vi "CODMn质控流程 (子VI).vi"(9 "CODMn量程切换":enum32{"H", "L", "AUTO"}(ring)=enum."AUTO", 10 "CODMn":bool) -> (3 "布尔":bool)   [LabVIEW 2016, in "质控单元.lvlib"]
panel:
  out "CODMn中断报警":bool
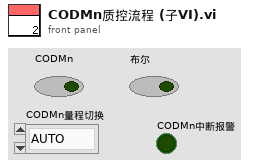
[diagram p1: front panel]
types:
  T1 = enum16{"待机", "启动水样测量", "水样测量中", "启动加标", "启动加标回收", "加标回收测量中", "结束"}
  T2 = cluster{"测量模式":enum16{"水样测量", "标样核查", "零点核查", "跨度核查", "空白测试", "加标回收", "平行样", "校零", "校标"}}
  T3 = enum16{"空闲", "水样测试", "标样核查", "零点核查", "跨度核查", "空白测试", "平行样测试", "质控样", "空白校准", "标样校准", "加标回收"}
  T4 = enum16{"空闲", "水样测试", "标样核查", "零点核查", "跨度核查", "空白测试", "平行样测试", "加标回收", "空白校准", "标样校准", "初始化（清洗）"}
  T5 = cluster{"量程":dbl, "检出限":dbl, "加标前水样浓度":dbl, "加标后水样浓度":dbl, "加标水杯定容体积":dbl, "加标母液浓度":dbl, "加标体积":dbl, "加标回收率":dbl}
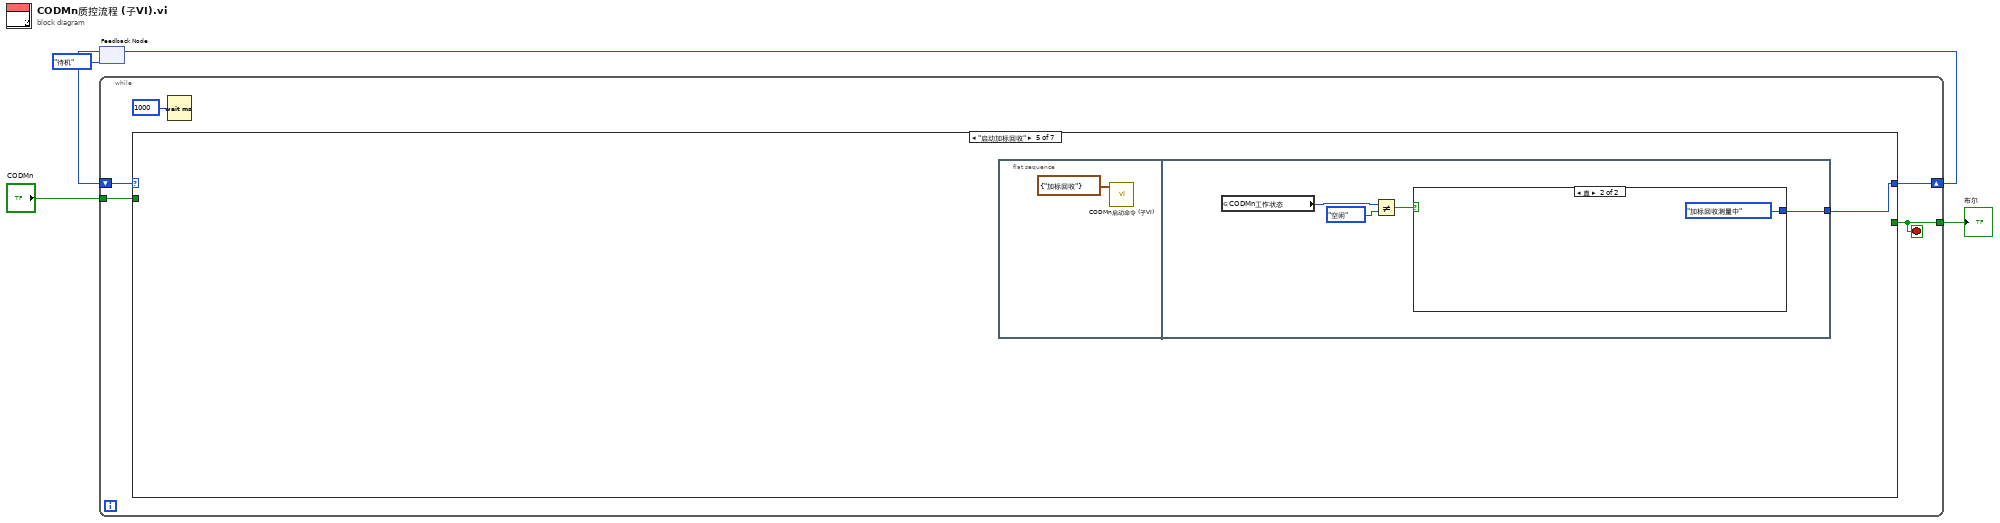
[diagram p0: block diagram]
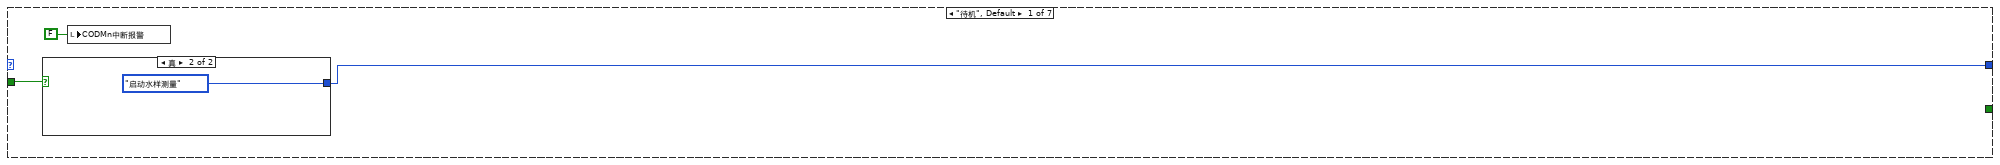
[diagram p2: hidden frame]
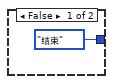
[diagram p3: hidden frame]
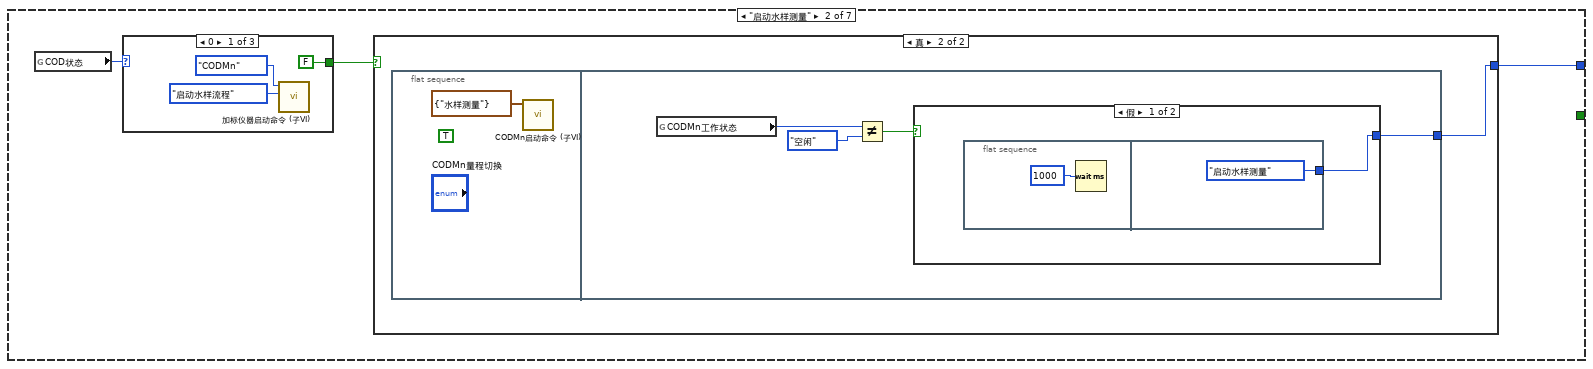
[diagram p4: hidden frame]
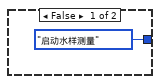
[diagram p5: hidden frame]
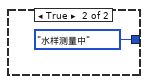
[diagram p6: hidden frame]
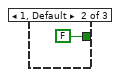
[diagram p7: hidden frame]
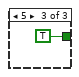
[diagram p8: hidden frame]
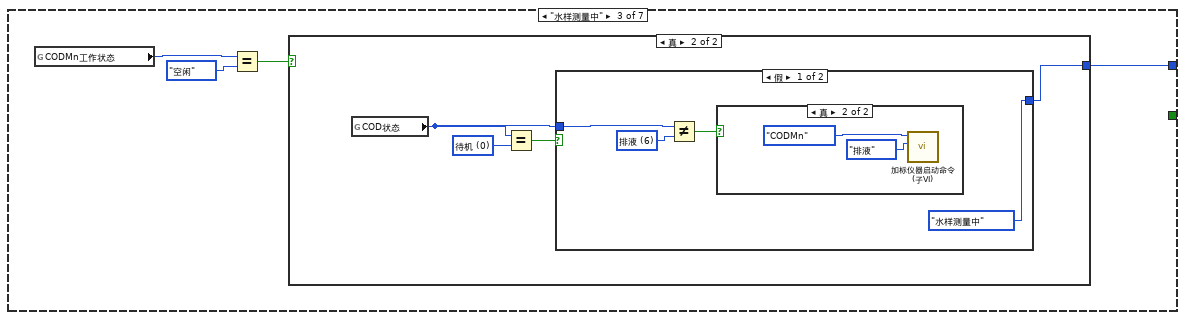
[diagram p9: hidden frame]
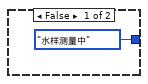
[diagram p10: hidden frame]
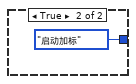
[diagram p12: hidden frame]
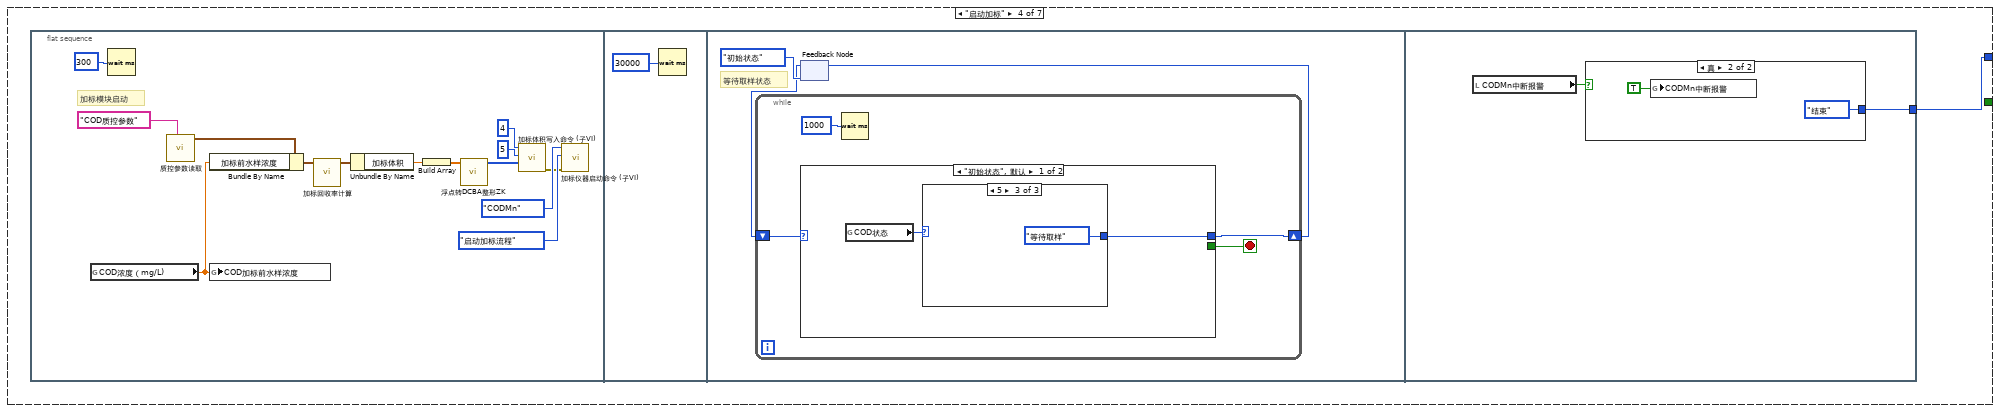
[diagram p13: hidden frame]
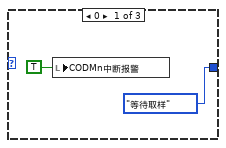
[diagram p14: hidden frame]
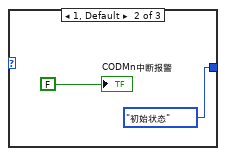
[diagram p15: hidden frame]
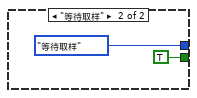
[diagram p16: hidden frame]
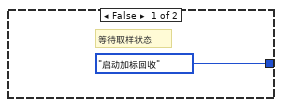
[diagram p17: hidden frame]
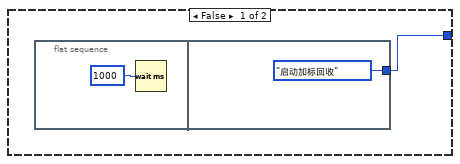
[diagram p18: hidden frame]
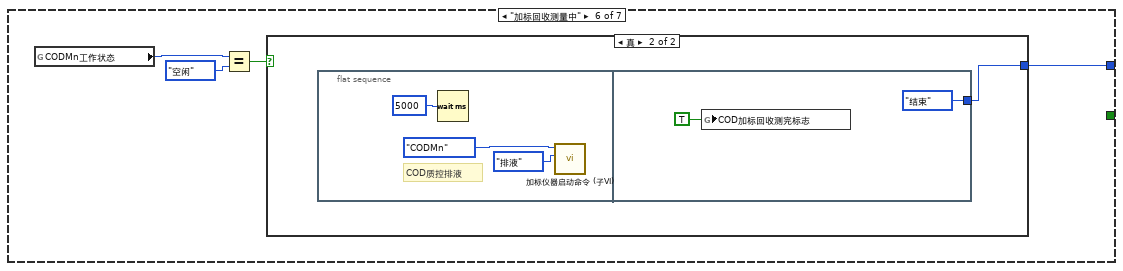
[diagram p19: hidden frame]
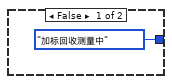
[diagram p20: hidden frame]
diagram:
  n1 = feedback #1(T1."待机") -> (w1:T1)
  n2 = while {
    tunnel: "CODMn" -> [w10]
    tunnel: [w6] -> w3
    shift-right: [w9] -> w4
    shift-left: w1 -> [w8]
    stop <- w6 stop-if-true
    n3 = case shown="\"启动加标回收\"" w8 {
      tunnel: [w13 w18 w38 w51 w88 w101 T1."结束"] -> w9
      tunnel: [_ _ _ _ _ _ TRUE] -> w6
      tunnel: w10 -> [w12 _ _ _ _ _ _]
      frame "待机", Default {
        n4 = case shown="真" w12 {
          tunnel: [T1."结束" T1."启动水样测量"] -> w13
          frame False {
          }
          frame True {
          }
        }
        n5 = local write "CODMn中断报警"(FALSE ("CODMn中断报警")) -> ()
      }
      frame "启动水样测量" {
        n6 = global read "加标回收状态全局变量.vi" "COD状态"() -> (w17:u16)
        n7 = case shown="0" w17 {
          tunnel: [FALSE ("s") FALSE ("s") TRUE ("s")] -> w16
          frame 0 {
            n8 = call "加标仪器启动命令 (子VI).vi"("启动命令"=enum16{"启动水样流程", "启动加标流程", "排液", "停止"}."启动水样流程", "仪器"=enum16{"", "氨氮", "总磷", "总氮", "CODMn", "CODCr"}."CODMn") -> ()  [unwired: 9 in, 1 out]
          }
          frame 1, Default {
          }
          frame 5 {
          }
        }
        n9 = case shown="真" w16 {
          tunnel: [T1."启动水样测量" w20] -> w18
          frame False {
          }
          frame True {
            n10 = flat-sequence {
              tunnel: [w25] -> w20
              frame #0 {
                (unwired) TRUE ("强制切换")
                n11 = call "CODMn启动命令 (子VI).vi"("启动测量模式"=T2 {"测量模式"=enum."水样测量"}) -> ()  [unwired: 10 in, 1 out]
              }
              frame #1 {
                n12 = global read "与CODMn交互全局.vi" "CODMn工作状态"() -> (w24:T4)
                n13 = Not Equal?(x=w24, y=T3."空闲") -> (x != y?=w22:bool)
                n14 = case shown="假" w22 {
                  tunnel: [w26 T1."水样测量中"] -> w25
                  frame False {
                    n15 = flat-sequence {
                      tunnel: [T1."启动水样测量"] -> w26
                      frame #0 {
                        n16 = Wait (ms)(milliseconds to wait=u32 1000 ("等待时间（毫秒）")) -> ()  [unwired: 1 out]
                      }
                      frame #1 {
                      }
                    }
                  }
                  frame True {
                  }
                }
              }
            }
          }
        }
      }
      frame "水样测量中" {
        n17 = global read "与CODMn交互全局.vi" "CODMn工作状态"() -> (w37:T4)
        n18 = Equal?(x=w37, y=T3."空闲") -> (x = y?=w35:bool)
        n19 = case shown="真" w35 {
          tunnel: [T1."水样测量中" w43] -> w38
          frame False {
          }
          frame True {
            w42 = u16 0 items=["待机", "润洗", "进样", "进样完成", "柱塞泵加标", "等待取液", "排液"] ("COD状态")
            n20 = global read "加标回收状态全局变量.vi" "COD状态"() -> (w40:u16)
            n21 = Equal?(x=w40, y=w42) -> (x = y?=w41:bool)
            n22 = case shown="假" w41 {
              tunnel: [T1."水样测量中" T1."启动加标"] -> w43
              tunnel: w40 -> [w45 _]
              frame False {
                w46 = u16 6 items=["待机", "润洗", "进样", "进样完成", "柱塞泵加标", "等待取液", "排液"] ("氨氮状态")
                n23 = Not Equal?(x=w45, y=w46) -> (x != y?=w44:bool)
                n24 = case shown="真" w44 {
                  frame False {
                  }
                  frame True {
                    n25 = call "加标仪器启动命令 (子VI).vi"("启动命令"=enum16{"启动水样流程", "启动加标流程", "排液", "停止"}."排液", "仪器"=enum16{"", "氨氮", "总磷", "总氮", "CODMn", "CODCr"}."CODMn") -> ()  [unwired: 9 in, 1 out]
                  }
                }
              }
              frame True {
              }
            }
          }
        }
      }
      frame "启动加标" {
        n26 = flat-sequence {
          tunnel: [w84] -> w51
          frame #0 {
            # "加标模块启动"
            n27 = global read "与CODMn交互全局.vi" "COD浓度（mg/L)"() -> (w60:dbl)
            n28 = Wait (ms)(milliseconds to wait=u32 300 ("等待时间（毫秒）")) -> ()  [unwired: 1 out]
            n29 = call "质控参数读取.vi"("section"="COD质控参数") -> ("参数"=w63:T5)  [unwired: 9 in, 1 out]
            n30 = Bundle By Name(cluster=w63, "加标前水样浓度"=w60) -> (w64:T5)
            n31 = global write "水样浓度全局.vi" "COD加标前水样浓度"(w60) -> ()
            n32 = call "加标回收率计算.vi"("参数"=w64) -> ("参数 out"=w62:T5)  [unwired: 9 in, 1 out]
            n33 = Unbundle By Name(w62) -> ("加标体积"=w61:dbl)
            n34 = Build Array(w61) -> (w58:dbl[])
            n35 = call "浮点转DCBA整形ZK.vi"("浮点数"=w58) -> ("DCBA整形输出"=w53:u16[])  [unwired: 10 in]
            n36 = call "加标体积写入命令 (子VI).vi"("values"=w53, "starting address"=u16 5, "Slave ID"=u16 4 ("value")) -> ("错误输出"=w52:errorcluster)  [unwired: 8 in]
            n37 = call "加标仪器启动命令 (子VI).vi"("错误输入（无错误）"=w52, "启动命令"=enum16{"启动水样流程", "启动加标流程", "排液", "停止"}."启动加标流程", "仪器"=enum16{"", "氨氮", "总磷", "总氮", "CODMn", "CODCr"}."CODMn") -> ()  [unwired: 8 in, 1 out]
          }
          frame #1 {
            n38 = Wait (ms)(milliseconds to wait=u32 30000 ("等待时间（毫秒）")) -> ()  [unwired: 1 out]
          }
          frame #2 {
            # "等待取样状态"
            n39 = feedback #2(enum16{"初始状态", "等待取样"}."初始状态") -> (w68:enum16{"初始状态", "等待取样"})
            n40 = while {
              shift-right: [w72] -> w67
              shift-left: w68 -> [w73]
              stop <- w71 stop-if-true
              n41 = case shown="\"初始状态\", 默认" w73 {
                tunnel: [w75 enum16{"初始状态", "等待取样"}."等待取样"] -> w72
                tunnel: [_ TRUE] -> w71
                frame "初始状态", Default {
                  n42 = global read "加标回收状态全局变量.vi" "COD状态"() -> (w74:u16)
                  n43 = case shown="5" w74 {
                    tunnel: [enum16{"初始状态", "等待取样"}."等待取样" enum16{"初始状态", "等待取样"}."初始状态" enum16{"初始状态", "等待取样"}."等待取样"] -> w75
                    frame 0 {
                      n44 = local write "CODMn中断报警"(TRUE ("氨氮中断报警")) -> ()
                    }
                    frame 1, Default {
                      "CODMn中断报警" <- FALSE ("总氮中断报警")
                    }
                    frame 5 {
                    }
                  }
                }
                frame "等待取样" {
                }
              }
              n45 = Wait (ms)(milliseconds to wait=u32 1000 ("等待时间（毫秒）")) -> ()  [unwired: 1 out]
            }
            n46 = feedback-in #2(w67) -> ()
          }
          frame #3 {
            n47 = local read "CODMn中断报警"() -> (w83:bool)
            n48 = case shown="真" w83 {
              tunnel: [T1."启动加标回收" T1."结束"] -> w84
              frame False {
                # "等待取样状态"
              }
              frame True {
                n49 = global write "质控中断报警全局.vi" "CODMn中断报警"(TRUE ("CODMn中断报警")) -> ()
              }
            }
          }
        }
      }
      frame "启动加标回收" {
        n50 = flat-sequence {
          tunnel: [w93] -> w88
          frame #0 {
            n51 = call "CODMn启动命令 (子VI).vi"("启动测量模式"=T2 {"测量模式"=enum."加标回收"}) -> ()  [unwired: 10 in, 1 out]
          }
          frame #1 {
            n52 = global read "与CODMn交互全局.vi" "CODMn工作状态"() -> (w92:T4)
            n53 = Not Equal?(x=w92, y=T3."空闲") -> (x != y?=w90:bool)
            n54 = case shown="真" w90 {
              tunnel: [w94 T1."加标回收测量中"] -> w93
              frame False {
                n55 = flat-sequence {
                  tunnel: [T1."启动加标回收"] -> w94
                  frame #0 {
                    n56 = Wait (ms)(milliseconds to wait=u32 1000 ("等待时间（毫秒）")) -> ()  [unwired: 1 out]
                  }
                  frame #1 {
                  }
                }
              }
              frame True {
              }
            }
          }
        }
      }
      frame "加标回收测量中" {
        n57 = global read "与CODMn交互全局.vi" "CODMn工作状态"() -> (w100:T4)
        n58 = Equal?(x=w100, y=T3."空闲") -> (x = y?=w98:bool)
        n59 = case shown="真" w98 {
          tunnel: [T1."加标回收测量中" w103] -> w101
          frame False {
          }
          frame True {
            n60 = flat-sequence {
              tunnel: [T1."结束"] -> w103
              frame #0 {
                # "COD质控排液"
                n61 = Wait (ms)(milliseconds to wait=u32 5000 ("等待时间（毫秒）")) -> ()  [unwired: 1 out]
                n62 = call "加标仪器启动命令 (子VI).vi"("启动命令"=enum16{"启动水样流程", "启动加标流程", "排液", "停止"}."排液", "仪器"=enum16{"", "氨氮", "总磷", "总氮", "CODMn", "CODCr"}."CODMn") -> ()  [unwired: 9 in, 1 out]
              }
              frame #1 {
                n63 = global write "质控测完标志全局 1.vi" "COD加标回收测完标志"(TRUE ("COD加标回收测完标志")) -> ()
              }
            }
          }
        }
      }
      frame "结束" {
        n64 = Wait (ms)(milliseconds to wait=u32 5000 ("等待时间（毫秒）")) -> ()  [unwired: 1 out]
      }
    }
    n65 = Wait (ms)(milliseconds to wait=u32 1000 ("等待时间（毫秒）")) -> ()  [unwired: 1 out]
  }
  "布尔" <- w3
  n66 = feedback-in #1(w4) -> ()
